vi "Stepping Y.vi"(7 "Microstep size":T1(ring), 8 "error in (no error)":errorcluster, 9 "Delay":u32=5, 10 "Direction":bool, 11 "Enable":bool) -> (0 "error out":errorcluster)   [LabVIEW 2017]
doc: "To control the corresponding stepper motor (Y -axis) to step for a number of steps inputted by user."
panel:
  # "- A pulse will be given to Step pin of A4988 everytime this VI is used.\n- Increases the Delay value will slow down the stepper motor.\n- Larger microstep size will increase the resolution, but will slow down \n   the stepper motor too."
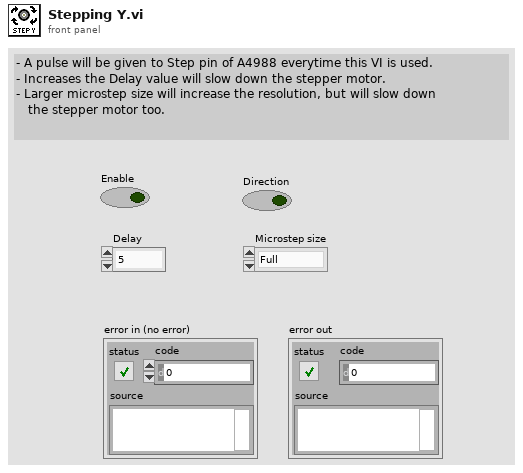
[diagram p1: front panel]
types:
  T1 = enum16{"Full", "Half", "Quarter", "Eighth", "Sixteenth"}
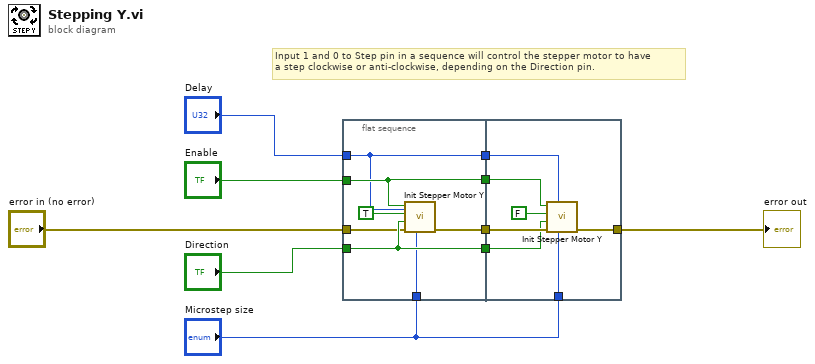
[diagram p0: block diagram]
diagram:
  # "Input 1 and 0 to Step pin in a sequence will control the stepper motor to have \na step clockwise or anti-clockwise, depending on the Direction pin."
  n1 = flat-sequence {
    tunnel: [w17] -> w10
    tunnel: "Enable" -> [w16]
    tunnel: [w16] -> w9
    tunnel: [w12] -> _
    tunnel: [w12] -> w8
    tunnel: "Direction" -> [w14]
    tunnel: [w14] -> w7
    tunnel: "Microstep size" -> [w13]
    tunnel: "Delay" -> [w12]
    tunnel: "error in (no error)" -> [w11]
    tunnel: w10 -> [w24]
    tunnel: w9 -> [w23]
    tunnel: w8 -> [w22]
    tunnel: w7 -> [w20]
    tunnel: "Microstep size" -> [w19]
    tunnel: [w18] -> w6
    frame #0 {
      n2 = call "Init Stepper Motor Y.vi"("Microstep size"=w13, "Delay"=w12, "error in (no error)"=w11, "Direction (A/DIO5 (Pin 21))"=w14, "Step (A/DIO4 (Pin 19))"=TRUE, "Enable (A/DIO0 (Pin 11))"=w16) -> ("error out"=w17:errorcluster)  [unwired: 5 in]
    }
    frame #1 {
      n3 = call "Init Stepper Motor Y.vi"("Microstep size"=w19, "Delay"=w22, "error in (no error)"=w24, "Direction (A/DIO5 (Pin 21))"=w20, "Step (A/DIO4 (Pin 19))"=FALSE, "Enable (A/DIO0 (Pin 11))"=w23) -> ("error out"=w18:errorcluster)  [unwired: 5 in]
    }
  }
  "error out" <- w6
